vi "Global Variable.vi"() -> ()   [LabVIEW 2016]
panel:
  out "Data":dbl
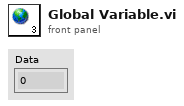
[diagram p1: front panel]
diagram:
